vi "main.vi"() -> ()   [LabVIEW 2016]
panel:
  out "X Home Position 2":string
  out "Y Home Position 2":string
  out "error out 4":errorcluster
  in  "error in 2":errorcluster
  out "Z Home Position 3":string
  out "Output status of pressure lines 2":bool[](array[boolean])
  out "error out 3":errorcluster
  in  "error in (no error)":errorcluster
  out "error out":errorcluster
  in  "error in":errorcluster
  out "X Axis Position 2":string
  out "Z Home Position 2":string
  out "Output status of pressure lines":bool[](array[boolean])
  out "error out 2":errorcluster
  in  "error in (no error) 2":errorcluster
  out "Z Incremental Position":string
  in  "stop":bool
  out "Z Axis Position":string
  out "X Absolute Positon":string
  out "Y Absolute Position":string
  out "X Home Position":string
  out "Y Home Position":string
  out "Z Home Position":string
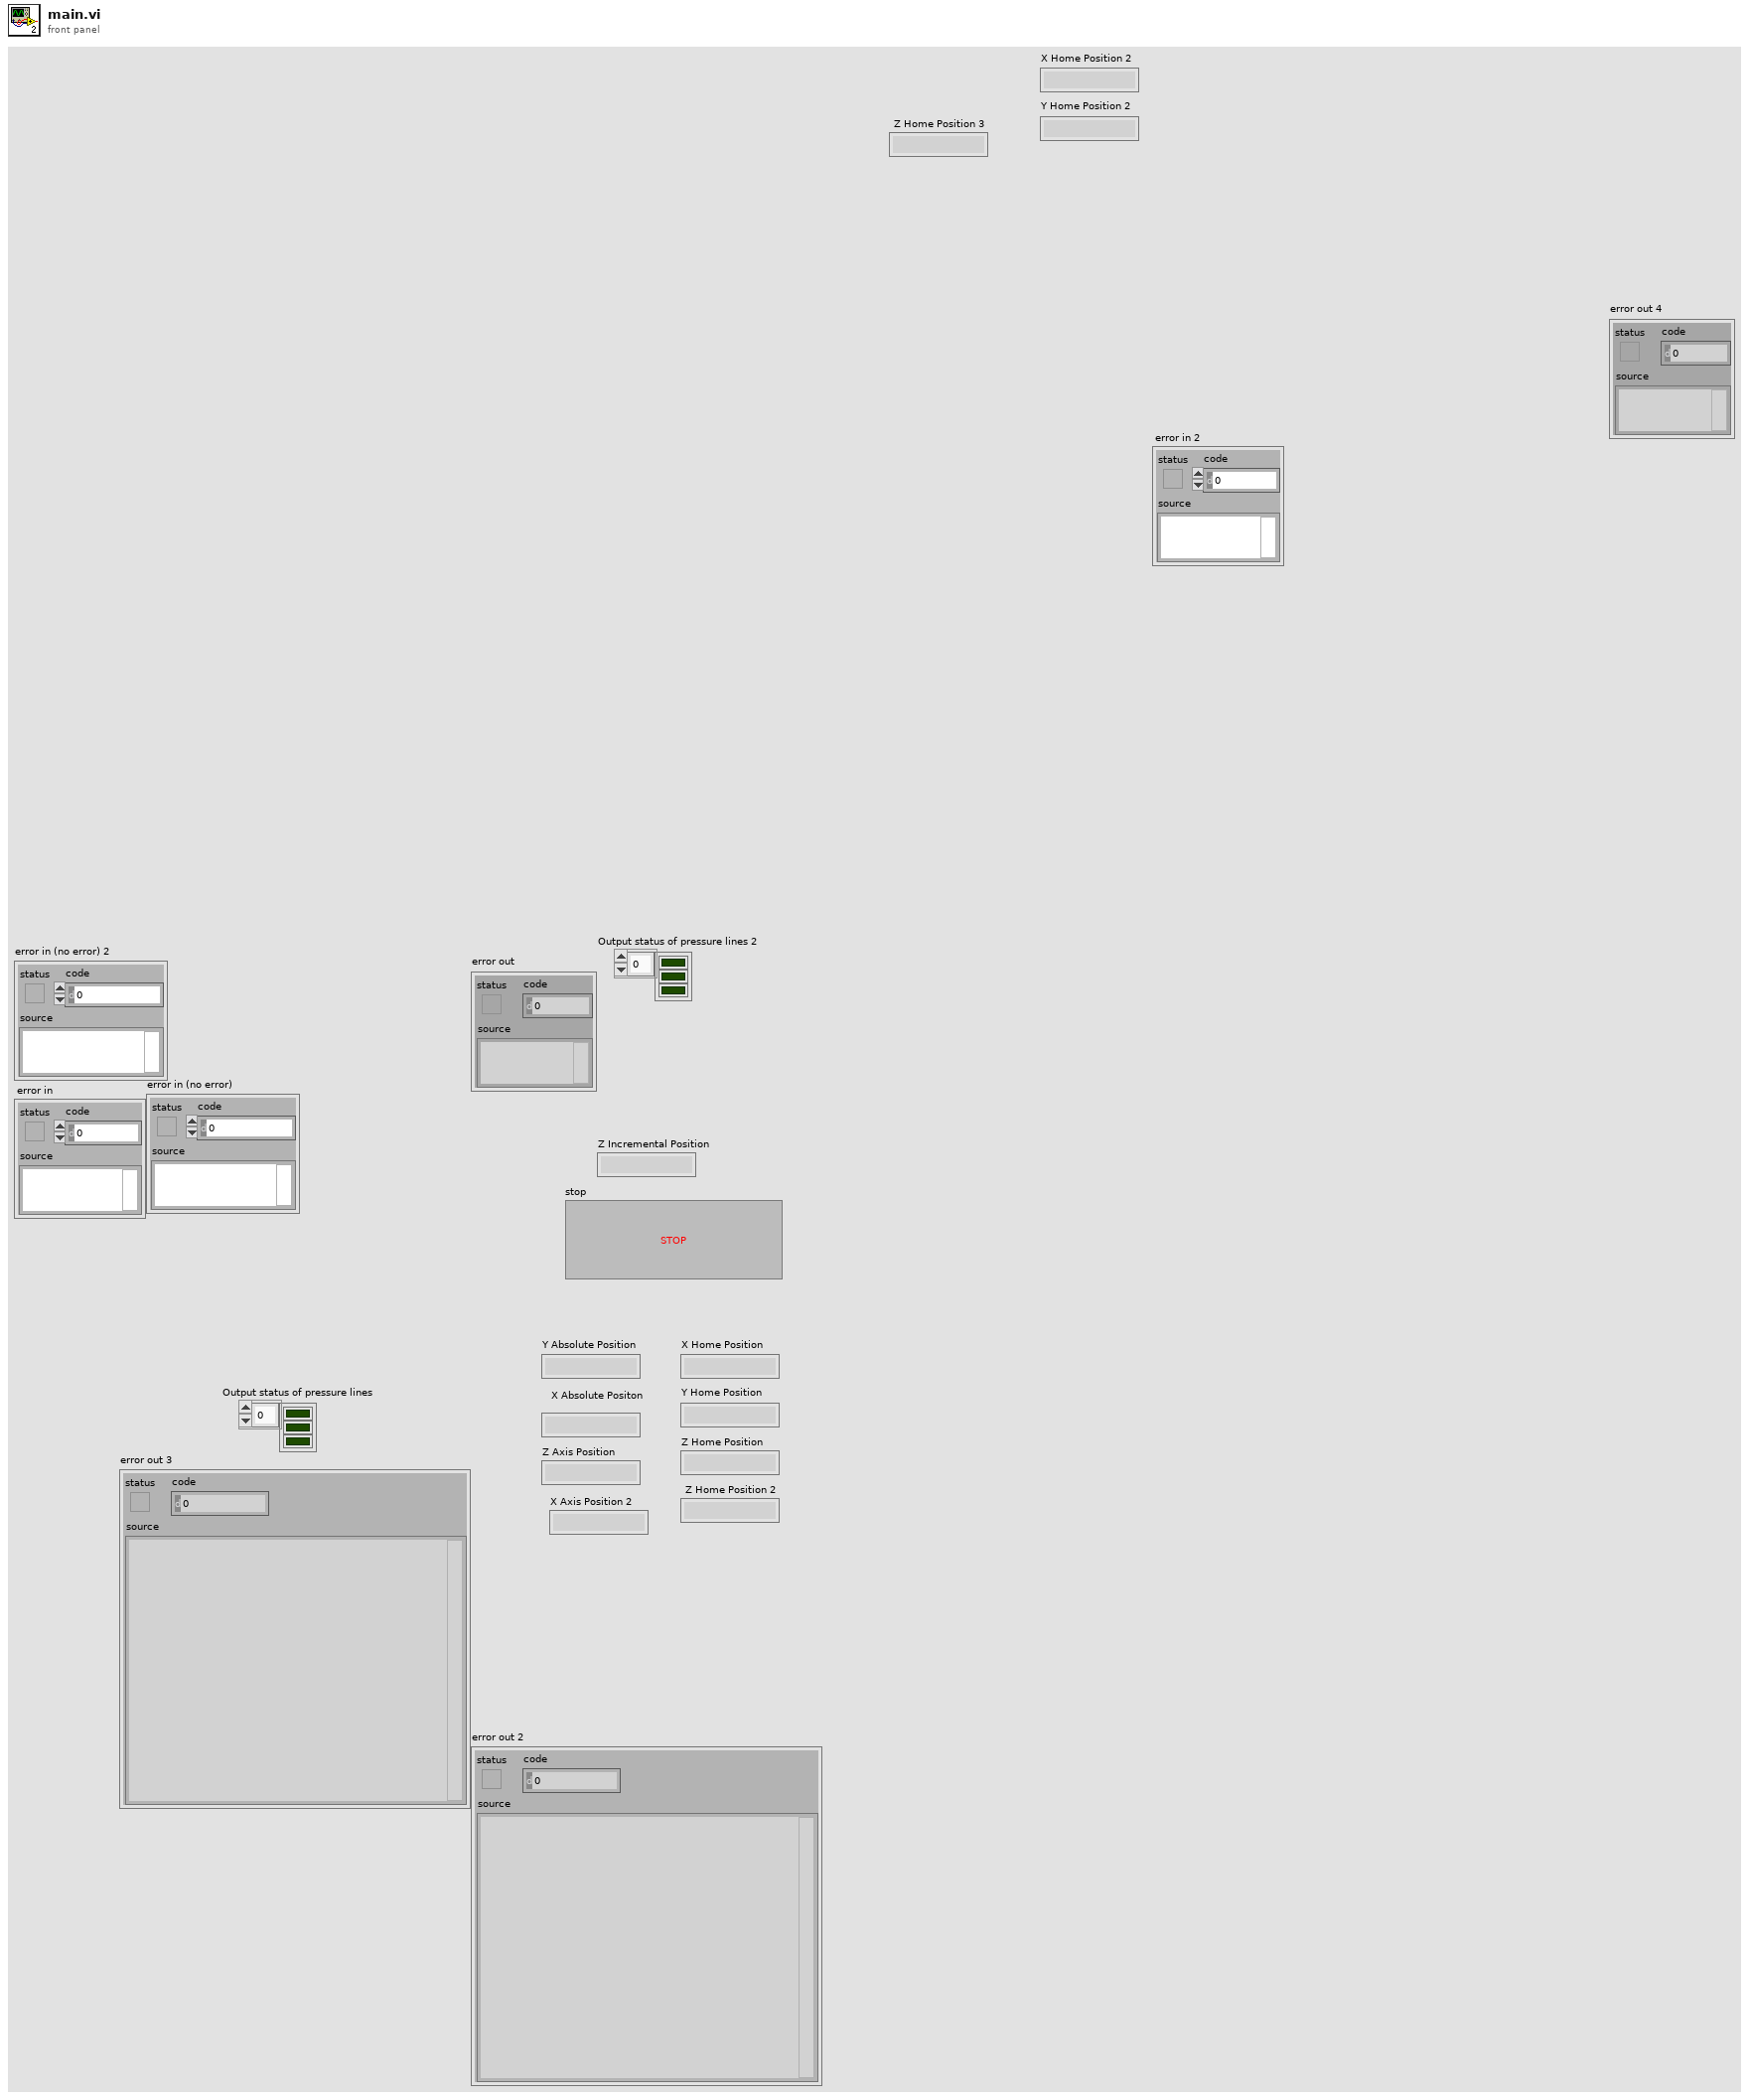
[diagram p1: front panel]
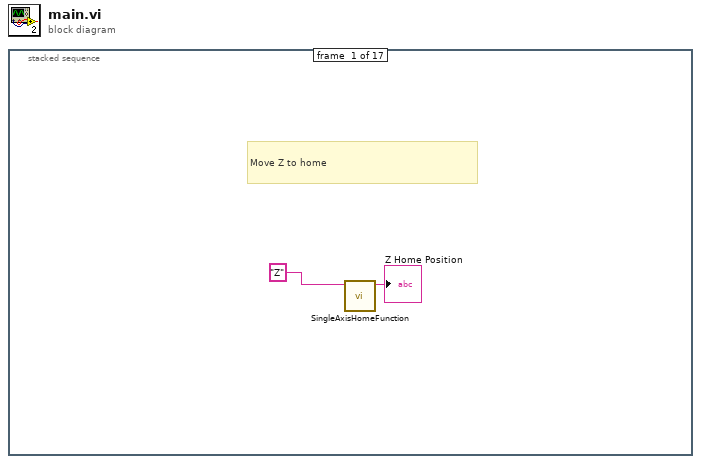
[diagram p0: block diagram]
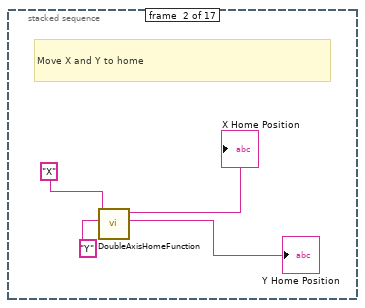
[diagram p2: hidden frame]
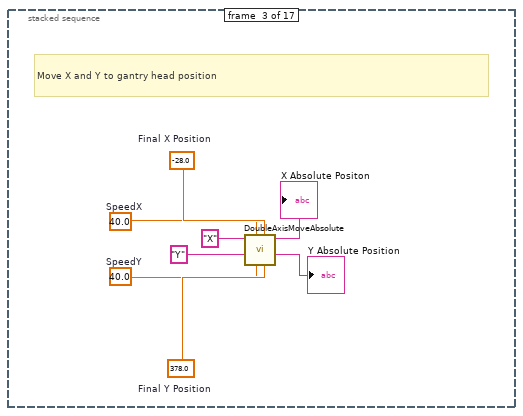
[diagram p3: hidden frame]
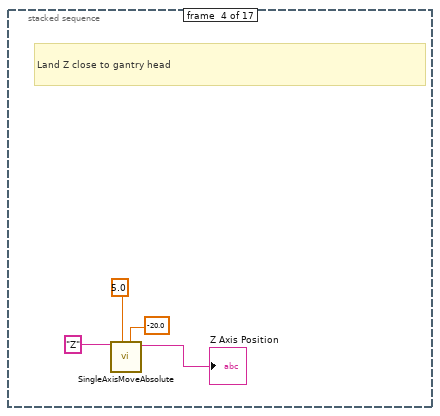
[diagram p4: hidden frame]
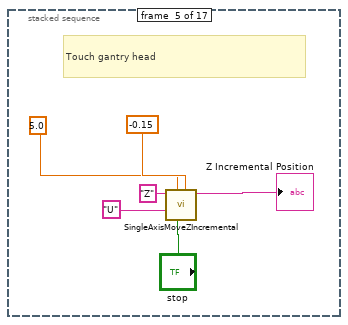
[diagram p5: hidden frame]
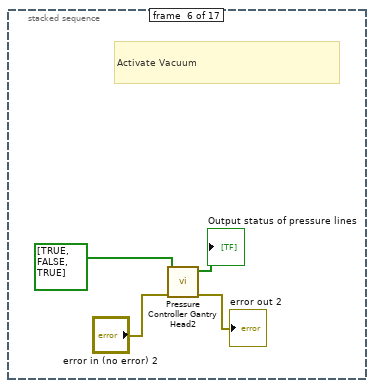
[diagram p6: hidden frame]
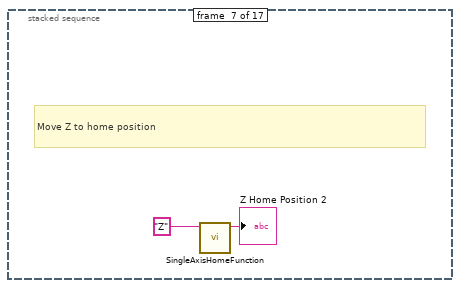
[diagram p7: hidden frame]
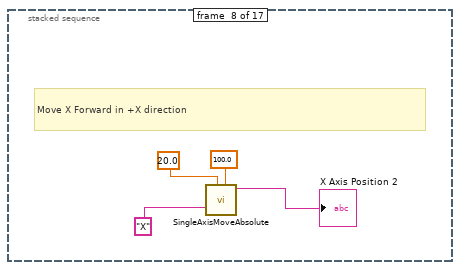
[diagram p8: hidden frame]
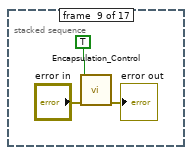
[diagram p9: hidden frame]
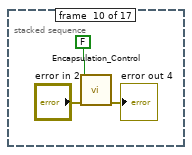
[diagram p10: hidden frame]
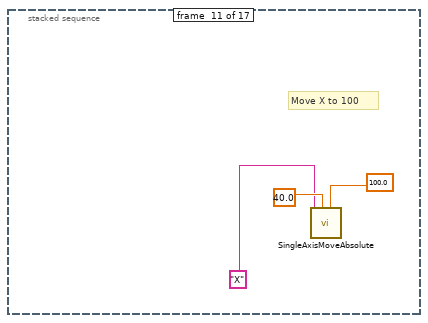
[diagram p11: hidden frame]
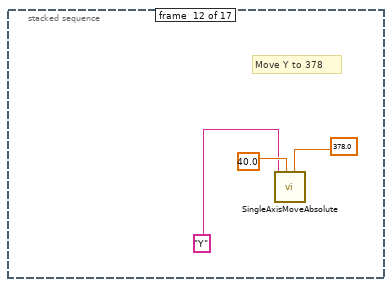
[diagram p12: hidden frame]
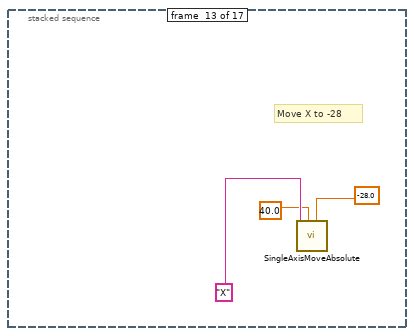
[diagram p13: hidden frame]
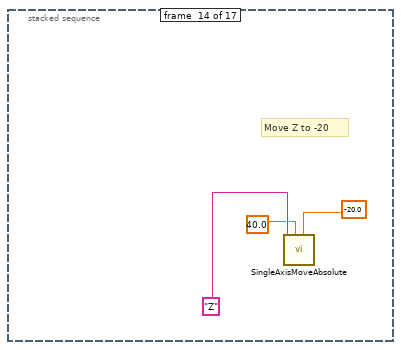
[diagram p14: hidden frame]
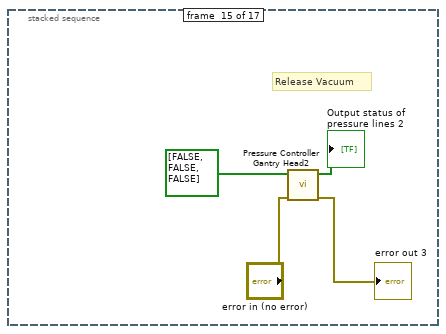
[diagram p15: hidden frame]
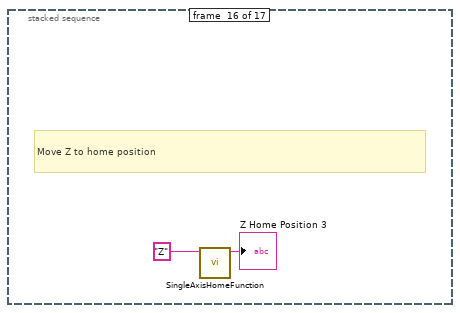
[diagram p16: hidden frame]
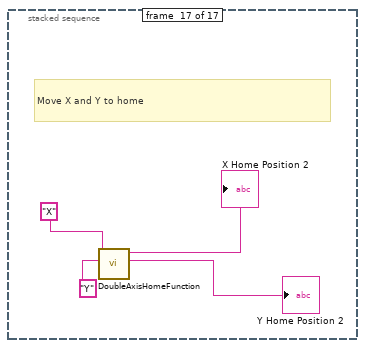
[diagram p17: hidden frame]
diagram:
  n1 = stacked-sequence {
    frame #0 {
      # "Move Z to home"
      n2 = call "SingleAxisHomeFunction.vi"("AxisName"="Z") -> ("Position"=→"Z Home Position":string)  [unwired: 10 in]
    }
    frame #1 {
      # "Move X and Y to home"
      n3 = call "DoubleAxisHomeFunction.vi"("Axis 2"="Y", "Axis 1"="X") -> ("Y Position"=→"Y Home Position":string, "X Position"=→"X Home Position":string)  [unwired: 8 in]
    }
    frame #2 {
      w12 = 40.0  # SpeedY
      w14 = 378.0  # Final Y Position
      w11 = 40.0  # SpeedX
      w13 = -28.0  # Final X Position
      # "Move X and Y to gantry head position"
      n4 = call "DoubleAxisMoveAbsolute.vi"("PositionY"=w14, "PositionX"=w13, "SpeedY"=w12, "SpeedX"=w11, "AxisName2"="Y", "AxisName1"="X") -> ("Y Absolute Position"=→"Y Absolute Position":string, "X Absolute Positon"=→"X Absolute Positon":string)  [unwired: 4 in]
    }
    frame #3 {
      # "Land Z close to gantry head"
      n5 = call "SingleAxisMoveAbsolute.vi"("Position"=-20.0, "Speed"=5.0, "AxisName"="Z") -> ("Axis Position"=→"Z Axis Position":string)  [unwired: 8 in]
    }
    frame #4 {
      # "Touch gantry head"
      n6 = call "SingleAxisMoveZIncremental.vi"("Distance"=-0.15, "stop"="stop", "Speed"=5.0, "\"FIX U\""="U" ("\"FIX U\""), "AxisName"="Z") -> ("Z Incremental Position"=→"Z Incremental Position":string)  [unwired: 6 in]
    }
    frame #5 {
      # "Activate Vacuum"
      n7 = call "Pressure Controller Gantry Head2.vi"("error in (no error)"="error in (no error) 2", "data"=bool[] [TRUE, FALSE, TRUE] ("data 2")) -> ("error out"=→"error out 2":errorcluster, "Output status of pressure lines"=→"Output status of pressure lines":bool[])  [unwired: 8 in]
    }
    frame #6 {
      # "Move Z to home position"
      n8 = call "SingleAxisHomeFunction.vi"("AxisName"="Z") -> ("Position"=→"Z Home Position 2":string)  [unwired: 10 in]
    }
    frame #7 {
      # "Move X Forward in +X direction"
      n9 = call "SingleAxisMoveAbsolute.vi"("Position"=100.0, "Speed"=20.0, "AxisName"="X") -> ("Axis Position"=→"X Axis Position 2":string)  [unwired: 8 in]
    }
    frame #8 {
      n10 = call "Encapsulation_Control.vi"("error in"="error in", "Encapsulation  State"=TRUE) -> ("error out"=→"error out":errorcluster)  [unwired: 9 in]
    }
    frame #9 {
      n11 = call "Encapsulation_Control.vi"("error in"="error in 2", "Encapsulation  State"=FALSE) -> ("error out"=→"error out 4":errorcluster)  [unwired: 9 in]
    }
    frame #10 {
      # "Move X to 100"
      n12 = call "SingleAxisMoveAbsolute.vi"("Position"=100.0, "Speed"=40.0, "AxisName"="X") -> ()  [unwired: 8 in, 1 out]
    }
    frame #11 {
      # "Move Y to 378"
      n13 = call "SingleAxisMoveAbsolute.vi"("Position"=378.0, "Speed"=40.0, "AxisName"="Y") -> ()  [unwired: 8 in, 1 out]
    }
    frame #12 {
      # "Move X to -28"
      n14 = call "SingleAxisMoveAbsolute.vi"("Position"=-28.0, "Speed"=40.0, "AxisName"="X") -> ()  [unwired: 8 in, 1 out]
    }
    frame #13 {
      # "Move Z to -20"
      n15 = call "SingleAxisMoveAbsolute.vi"("Position"=-20.0, "Speed"=40.0, "AxisName"="Z") -> ()  [unwired: 8 in, 1 out]
    }
    frame #14 {
      # "Release Vacuum"
      n16 = call "Pressure Controller Gantry Head2.vi"("error in (no error)"="error in (no error)", "data"=bool[] [FALSE, FALSE, FALSE]) -> ("error out"=→"error out 3":errorcluster, "Output status of pressure lines"=→"Output status of pressure lines 2":bool[])  [unwired: 8 in]
    }
    frame #15 {
      # "Move Z to home position"
      n17 = call "SingleAxisHomeFunction.vi"("AxisName"="Z") -> ("Position"=→"Z Home Position 3":string)  [unwired: 10 in]
    }
    frame #16 {
      # "Move X and Y to home"
      n18 = call "DoubleAxisHomeFunction.vi"("Axis 2"="Y", "Axis 1"="X") -> ("Y Position"=→"Y Home Position 2":string, "X Position"=→"X Home Position 2":string)  [unwired: 8 in]
    }
  }
